vi "Calc Eval.vi"(8 "error in (no error)":errorcluster, 10 "Inputs":dbl[](array[numeric]), 11 "Min Calc in":refnum<class "Min Calc.lvclass">) -> (0 "error out":errorcluster, 1 "Additional Updates":T1[](array[typedef]), 2 "Result":dbl, 3 "Min Calc out":refnum<class "Min Calc.lvclass">)   [LabVIEW 2020, in "VolatusCalcs.lvlib" / "Min Calc.lvclass"]
uses:
  Min Calc.lvclass
  Min Calc.lvclass/Min Calc.ctl
  Calculation/Additional Update.ctl
  Calculation/Calculation.lvclass
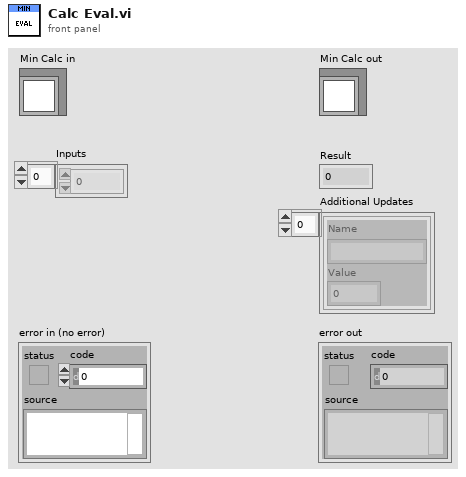
[diagram p1: front panel]
types:
  T1 = typedef "VolatusCalcs.lvlib/Calculation.lvclass/Additional Update.ctl" = cluster{"Name":string, "Value":dbl}
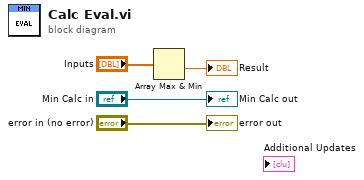
[diagram p0: block diagram]
diagram:
  n1 = Array Max & Min(array="Inputs") -> (min value=→"Result":dbl)  [unwired: 3 out]
  "error out" <- "error in (no error)"
  "Min Calc out" <- "Min Calc in"
